vi "Append Block Diagram Image.vi"(0 "PDF Report IN":refnum<class "PDF Report Class.lvclass">, 1 "Image size":T1={"Maximum Width"=-1, "Maximum Height"=-1}, 2 "Scale (%)":sgl=100.0, 3 "Border":T2={"Show?"=FALSE, "Thickness (point)"=0.5, "Color"=0}, 5 "VI reference":refnum<vi>, 11 "error in (no error)":errorcluster, 12 "Caption":string, 14 "Position and indentation":T3={"Alignment"=enum."Center", "X "=0.0, "Y"=0.0, "Indentation"=0.0}) -> (4 "PDF Report OUT":refnum<class "PDF Report Class.lvclass">, 15 "error out":errorcluster)   [LabVIEW 2019]
doc: "Creates an image of the block diagram of the VI you specify in <B>VI reference</B> and appends it to a PDF report. <B>Not Available in Run-Time </B>.\n\n<B>FRANÇAIS</B>\nCréation de l'image du \"block diagram\" que vous avez spécifié par <B>VI reference</B> et ajout au rapport PDF. <B>Ce VI fonctionne uniquement en mode développement</B>.\n\nVersion 1.0\nDeveloped by Jean-Marc Simard\nCopyright © 2010, Exaprom Inc.\nAll rights reserved.\nLicense: BSD\n\nWith iTextSharp 4.1.6 (http://itextsharp.sourceforge.net)\nunder Mozilla Public License Version 1.1\n(http://www.mozilla.org/MPL/MPL-1.1.html)"
uses:
  <userlib>/Exaprom PDF/LV Class/PDF Report Class/PDF Report Class.lvclass
  <userlib>/Exaprom PDF/Controls/Image Controls/Image alignment and position.ctl
  <userlib>/Exaprom PDF/Controls/Image Controls/Image aligment.ctl
  <userlib>/Exaprom PDF/Controls/Image Controls/Image border.ctl
  <userlib>/Exaprom PDF/Controls/Image Controls/Image Size Block Diagram.ctl
  <userlib>/Exaprom PDF/Controls/Font Controls/Font complete cluster.ctl
  <userlib>/Exaprom PDF/Controls/Font Controls/Font size.ctl
  <userlib>/Exaprom PDF/Controls/Font Controls/Font color.ctl
  <userlib>/Exaprom PDF/Controls/Font Controls/Type and encoding.ctl
  <userlib>/Exaprom PDF/Controls/Text Controls/Unicode/Type and run direction.ctl
  C:/Program Files/National Instruments/LabVIEW 2019/user.lib/Exaprom PDF/DLL/itextsharp.dll
  DLL/itextsharp.dll
panel:
  out "Size (points)":cluster{"TotalHeight":sgl, "TotalWidth":sgl}
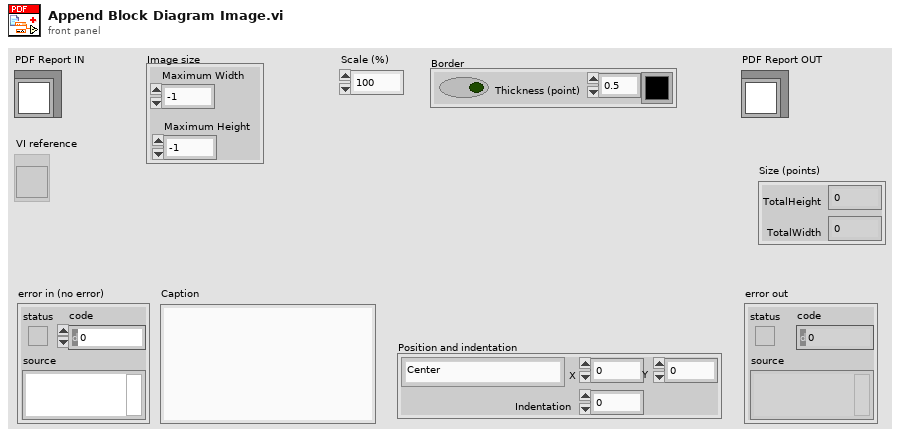
[diagram p1: front panel]
types:
  T1 = typedef "Image Size Block Diagram.ctl" = cluster{"Maximum Width":i32, "Maximum Height":i32}
  T2 = typedef "Image border.ctl" = cluster{"Show?":bool, "Thickness (point)":sgl, "Color":u32}
  T3 = typedef "Image alignment and position.ctl" = cluster{"Alignment":T4, "X ":sgl, "Y":sgl, "Indentation":sgl}
  T4 = typedef "Image aligment.ctl" = enum16{"Absolute (X,Y)", "Left", "Center", "Right", "Left (textwrap)", "Right (textwrap)"}
  T5 = typedef "Font complete cluster.ctl" = cluster{"Name":string, "Size":T6, "Color":T7, "Style":cluster{"Bold":bool, "Italic":bool, "Underline":bool, "Strikeout":bool}, "Type":T8}
  T6 = typedef "Font size.ctl" = sgl
  T7 = typedef "Font color.ctl" = u32
  T8 = typedef "Type and encoding.ctl" = cluster{"Type&direction":T9, "Embedded":bool, "Encoding":string}
  T9 = typedef "Type and run direction.ctl" = enum16{"Select", "ASCII", "UTF-16", "UTF-16 (default)", "UTF-16 (LTR)", "UTF-16 (RTL)"}
  T10 = enum32{"invalid app kind", "Development System", "Run Time System", "Student Edition", "Embedded LabVIEW", "Evaluation", "Custom"}
  T11 = typedef "imagedata.ctl" = cluster{"image type":i32, "image depth":i32, "image":u8[], "mask":u8[], "colors":u32[], "Rectangle":cluster{"left":i16, "top":i16, "right":i16, "bottom":i16}}
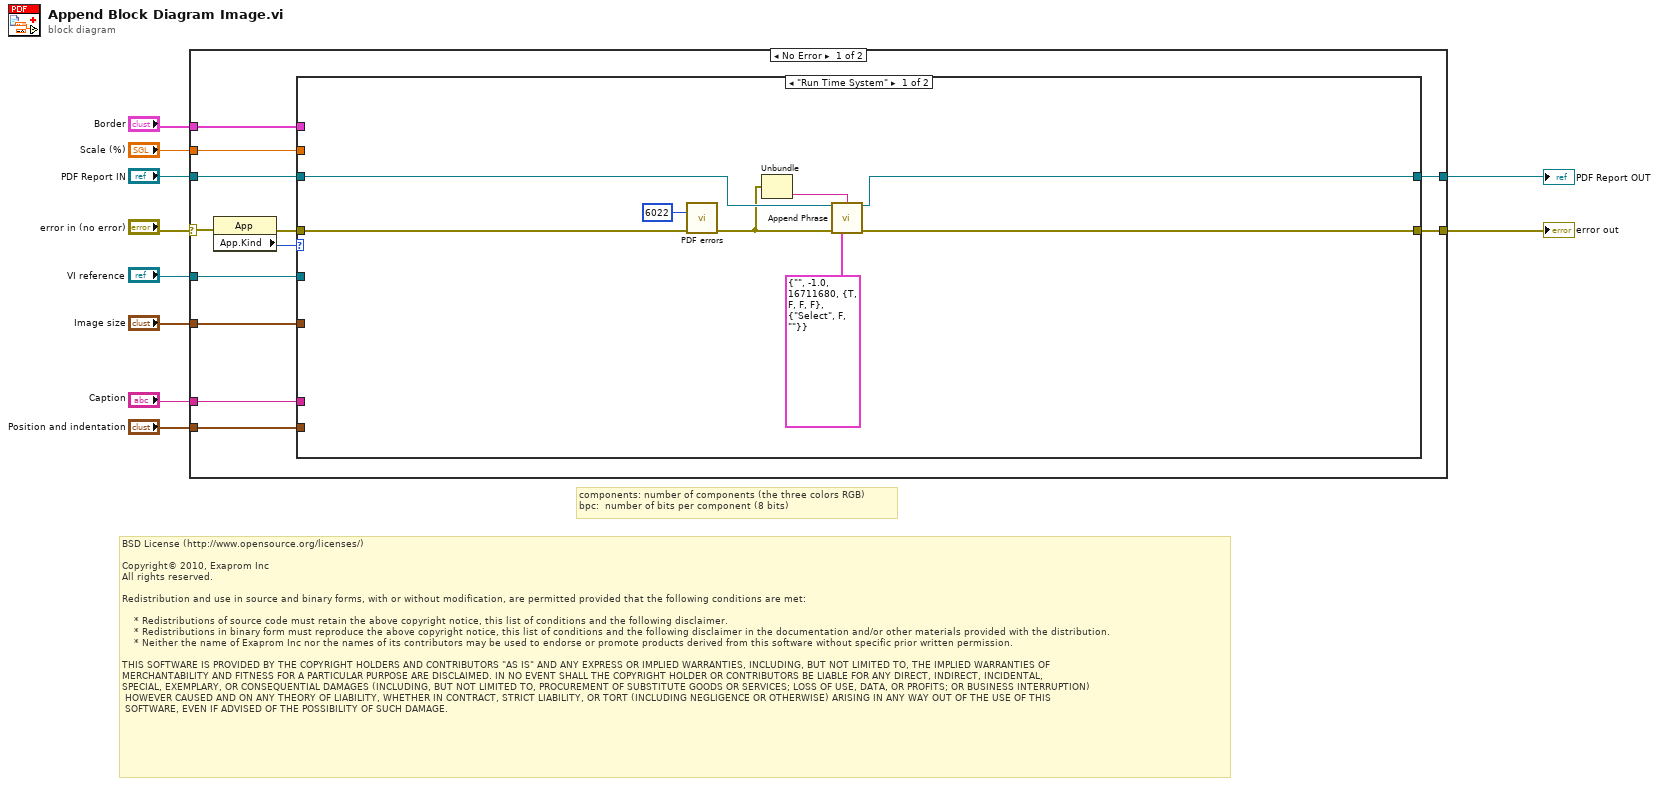
[diagram p0: block diagram]
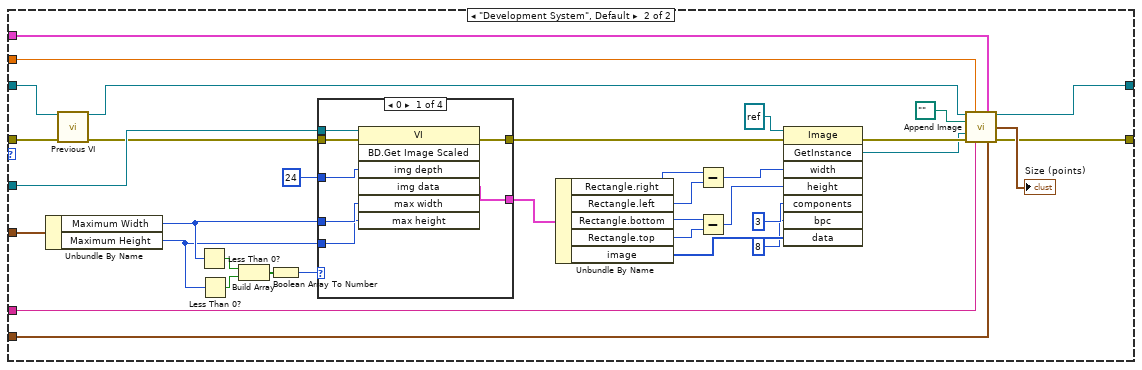
[diagram p2: hidden frame]
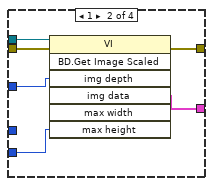
[diagram p3: hidden frame]
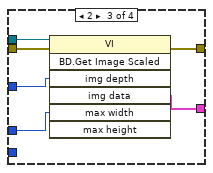
[diagram p4: hidden frame]
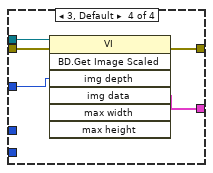
[diagram p5: hidden frame]
diagram:
  # "components: number of components (the three colors RGB)\nbpc:  number of bits per component (8 bits)"
  # "BSD License (http://www.opensource.org/licenses/)\n\nCopyright© 2010, Exaprom Inc\nAll rights reserved.\n\nRedistribution and use in source and binary forms, with or without modification, are permitted provided that the following conditions are met:\n\n    * Redistributions of source code must retain the above copyright notice, this list of conditions and the following disclaimer.\n    * Redistributions in binary form must reproduce the above copyright notice, this list of conditions and the following disclaimer in the documentation and/or other materials provided with the distribution.\n    * Neither the name of Exaprom Inc nor the names of its contributors may be used to endorse or promote products derived from this software without specific prior written permission.\n\nTHIS SOFTWARE IS PROVIDED BY THE COPYRIGHT HOLDERS AND CONTRIBUTORS \"AS IS\" AND ANY EXPRESS OR IMPLIED WARRANTIES, INCLUDING, BUT NOT LIMITED TO, THE IMPLIED WARRANTIES OF \nMERCHANTABILITY AND FITNESS FOR A PARTICULAR PURPOSE ARE DISCLAIMED. IN NO EVENT SHALL THE COPYRIGHT HOLDER OR CONTRIBUTORS BE LIABLE FOR ANY DIRECT, INDIRECT, INCIDENTAL,\nSPECIAL, EXEMPLARY, OR CONSEQUENTIAL DAMAGES (INCLUDING, BUT NOT LIMITED TO, PROCUREMENT OF SUBSTITUTE GOODS OR SERVICES; LOSS OF USE, DATA, OR PROFITS; OR BUSINESS INTERRUPTION)\n HOWEVER CAUSED AND ON ANY THEORY OF LIABILITY, WHETHER IN CONTRACT, STRICT LIABILITY, OR TORT (INCLUDING NEGLIGENCE OR OTHERWISE) ARISING IN ANY WAY OUT OF THE USE OF THIS\n SOFTWARE, EVEN IF ADVISED OF THE POSSIBILITY OF SUCH DAMAGE."
  n1 = case shown="No Error" "error in (no error)" {
    selector: "error in (no error)" -> [w11 w91]
    tunnel: [w19 w91] -> w3
    tunnel: "VI reference" -> [w22 _]
    tunnel: [w20 w90] -> w2
    tunnel: "PDF Report IN" -> [w21 w90]
    tunnel: "Caption" -> [w18 _]
    tunnel: "Position and indentation" -> [w17 _]
    tunnel: "Border" -> [w16 _]
    tunnel: "Scale (%)" -> [w15 _]
    tunnel: "Image size" -> [w14 _]
    frame No Error {
      n2 = property class="App"(error in=w11) -> (error out=w12:errorcluster, "App.Kind"=w13:T10)  [unwired: 1 in, 1 out]
      n3 = case shown="\"Run Time System\"" w13 {
        tunnel: w22 -> [_ w65]
        tunnel: w21 -> [w28 w62]
        tunnel: [w27 w31] -> w20
        tunnel: [w26 w32] -> w19
        tunnel: w18 -> [_ w61]
        tunnel: w17 -> [_ w60]
        tunnel: w16 -> [_ w59]
        tunnel: w15 -> [_ w58]
        tunnel: w12 -> [w30 w55]
        tunnel: w14 -> [_ w53]
        frame "Run Time System" {
          n4 = call <userlib>:"PDF errors.vi"("code"=6022, "error in (no error)"=w30) -> ("error out"=w25:errorcluster)  [unwired: 1 in, 12 out]
          n5 = Unbundle(w25) -> ("source"=w24:string)  [unwired: 2 out]
          n6 = call <userlib>:"Append Phrase.vi"("PDF Report IN"=w28, "Text"=w24, "error in (no error)"=w25, "Font"=T5 {"Name"="", "Size"=-1.0, "Color"=16711680, "Style"={"Bold"=TRUE, "Italic"=FALSE, "Underline"=FALSE, "Strikeout"=FALSE}, "Type"={"Type&direction"=enum."Select", "Embedded"=FALSE, "Encoding"=""}} ("Font complete")) -> ("PDF Report OUT"=w27:refnum<class "PDF Report Class.lvclass">, "error out"=w26:errorcluster)  [unwired: 1 in, 9 out]
        }
        frame "Development System", Default {
          n7 = Unbundle By Name(w53) -> ("Maximum Width"=w39:i32, "Maximum Height"=w38:i32)
          n8 = call <userlib>:"Previous VI.vi"("PDF Report IN"=w62, "error in (no error)"=w55) -> ("PDF Report OUT"=w33:refnum<class "PDF Report Class.lvclass">, "error out"=w54:errorcluster)  [unwired: 12 out]
          n9 = Less Than 0?(x=w39) -> (x < 0?=w37:bool)
          n10 = Less Than 0?(x=w38) -> (x < 0?=w36:bool)
          n11 = Build Array(w37, w36) -> (w35:bool[])
          n12 = Boolean Array To Number(Boolean array=w35) -> (number=w34:u32)
          n13 = case shown="0" w34 {
            tunnel: [w72 w78 w84 w89] -> w52
            tunnel: w65 -> [w71 w77 w83 w88]
            tunnel: [w70 w76 w82 w87] -> w41
            tunnel: 24 ("Image Depth") -> [w69 w75 w81 w86]
            tunnel: w54 -> [w68 w74 w80 w85]
            tunnel: w39 -> [w67 _ w79 _]
            tunnel: w38 -> [w66 w73 _ _]
            frame 0 {
              n14 = invoke class="VI" method="BD.Get Image Scaled"(reference=w71, error in=w68, "img depth"=w69, "max width"=w67, "max height"=w66) -> (error out=w72:errorcluster, "img data"=w70:T11)  [unwired: 2 in, 5 out]
            }
            frame 1 {
              n15 = invoke class="VI" method="BD.Get Image Scaled"(reference=w77, error in=w74, "img depth"=w75, "max height"=w73) -> (error out=w78:errorcluster, "img data"=w76:T11)  [unwired: 3 in, 5 out]
            }
            frame 2 {
              n16 = invoke class="VI" method="BD.Get Image Scaled"(reference=w83, error in=w80, "img depth"=w81, "max width"=w79) -> (error out=w84:errorcluster, "img data"=w82:T11)  [unwired: 3 in, 5 out]
            }
            frame 3, Default {
              n17 = invoke class="VI" method="BD.Get Image Scaled"(reference=w88, error in=w85, "img depth"=w86) -> (error out=w89:errorcluster, "img data"=w87:T11)  [unwired: 4 in, 5 out]
            }
          }
          n18 = Unbundle By Name(w41) -> ("Rectangle.right"=w50:i16, "Rectangle.left"=w49:i16, "Rectangle.bottom"=w47:i16, "Rectangle.top"=w46:i16, "image"=w43:u8[])
          n19 = Subtract(x=w50, y=w49) -> (x-y=w48:i16)
          n20 = Subtract(x=w47, y=w46) -> (x-y=w45:i16)
          n21 = invoke class="Image" method="GetInstance"(reference=refnum<k24> refnum ("image"), error in=w52, "width"=w48, "height"=w45, "components"=3, "bpc"=8, "data"=w43) -> (error out=w63:errorcluster, "GetInstance"=w57:refnum<k24>)  [unwired: 1 in, 6 out]
          n22 = call <userlib>:"Append Image.vi"("PDF Report IN"=w33, "Scale (%)"=w58, "Border"=w59, "Image path"=path "" ("path"), "Image Ref iTexSharp"=w57, "error in (no error)"=w63, "Caption"=w61, "Position and indentation"=w60) -> ("PDF Report OUT"=w31:refnum<class "PDF Report Class.lvclass">, "Size (points)"=→"Size (points)":cluster{"TotalHeight":sgl, "TotalWidth":sgl}, "error out"=w32:errorcluster)  [unwired: 5 out]
        }
      }
    }
    frame Error {
    }
  }
  "error out" <- w3
  "PDF Report OUT" <- w2
